vi "Extract_Country_Data.vi"(8 "Country":string, 11 "Raw Data Array (String)":string[][](array[string])) -> (3 "Country Data":string[][](array[string]))   [LabVIEW 2015]
doc: "This VI extracts all the instances of a particular country from the 2D-array of strings"
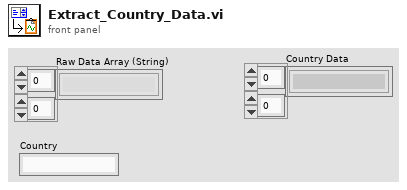
[diagram p1: front panel]
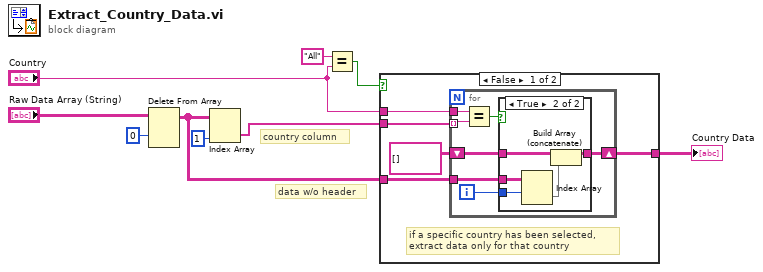
[diagram p0: block diagram]
diagram:
  # "country column"
  # "data w/o header"
  n1 = Delete From Array(array="Raw Data Array (String)", index (row)=0) -> (array with subset deleted=w5:string[][])  [unwired: 2 in, 1 out]
  n2 = Index Array(array=w5, index (col)=1 ("index (row)")) -> (element=w2:string[])  [unwired: 1 in]
  n3 = Equal?(x="All", y="Country") -> (x = y?=w4:bool)
  n4 = case shown="False" w4 {
    tunnel: w2 -> [w14 _]
    tunnel: "Country" -> [w13 _]
    tunnel: w5 -> [w12 w28]
    tunnel: [w10 w28] -> w6
    frame False {
      # "if a specific country has been selected, \nextract data only for that country"
      n5 = for {
        tunnel: w14 -> [w19] mode=indexing
        tunnel: w13 -> [w21]
        shift-right: [w18] -> w10
        shift-left: string[][] [] -> [w17]
        tunnel: w12 -> [w16]
        i -> [w15]
        n6 = Equal?(x=w21, y=w19) -> (x = y?=w20:bool)
        n7 = case shown="True" w20 {
          tunnel: w17 -> [w22 w27]
          tunnel: [w22 w26] -> w18
          tunnel: w16 -> [_ w25]
          tunnel: w15 -> [_ w24]
          frame False {
          }
          frame True {
            n8 = Index Array(array=w25, index (row)=w24) -> (element=w23:string[])  [unwired: 1 in]
            n9 = Build Array (concatenate)(w27, w23) -> (w26:string[][])
          }
        }
      }
    }
    frame True {
      # "all countries selected"
    }
  }
  "Country Data" <- w6
